vi "Get Device Name.vi"(8 "Error In":errorcluster, 11 "LINX Device Config":T1) -> (0 "Error Out":errorcluster, 2 "Device Name":string, 3 "LINX Device Config":T1)   [LabVIEW 2014, in "LMH-LINX.lvlib" / "Device.lvlib"]
uses:
  Device.lvlib
  Type Defs/LINX Device Config.ctl
  Type Defs/Interface.ctl
  Type Defs/TCP Config.ctl
  Type Defs/Channels.ctl
  Type Defs/Error Type.ctl
  LMH-LINX.lvlib
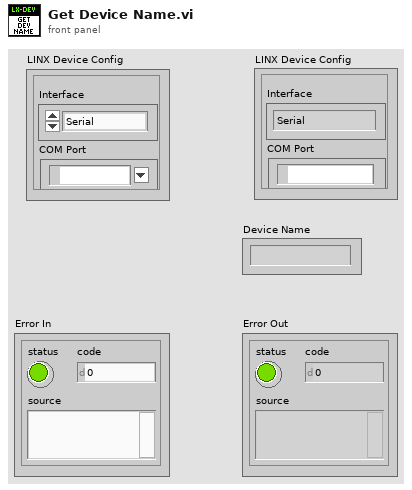
[diagram p1: front panel]
types:
  T1 = typedef "LMH-LINX.lvlib/Device.lvlib/LINX Device Config.ctl" = cluster{"Interface":T2, "COM Port":refnum<visa-resource-name>, "TCP Configuration":T3, "Device Family":u8, "Device ID":u8, "Device Name":string, "TCP Ref":refnum<k5>, "Channels":T4}
  T2 = typedef "LMH-LINX.lvlib/Interface.ctl" = enum16{"Serial", "TCP"}
  T3 = typedef "LMH-LINX.lvlib/Device.lvlib/TCP Config.ctl" = cluster{"IP Address":string, "Port":u16}
  T4 = typedef "LMH-LINX.lvlib/Channels.ctl" = cluster{"DI":u8[], "DO":u8[], "AI":u8[], "AO":u8[], "PWM":u8[], "QE":u8[], "UART":u8[], "I2C 2":u8[], "SPI":u8[], "CAN":u8[], "Servo":u8[], "AI Ref (V)":dbl, "AO Ref (V)":dbl, "AO Resolution (Bits)":u8}
  T5 = typedef "LMH-LINX.lvlib/Error Type.ctl" = enum16{"Unknown", "Timeout", "Corrupt Return Packet", "Unable To Connect", "Command Not Supported", "Channel DNE", "Invalid COM Config", "Firmware Version Mismatch", "myRIO Support", "CMD Specific Error"}
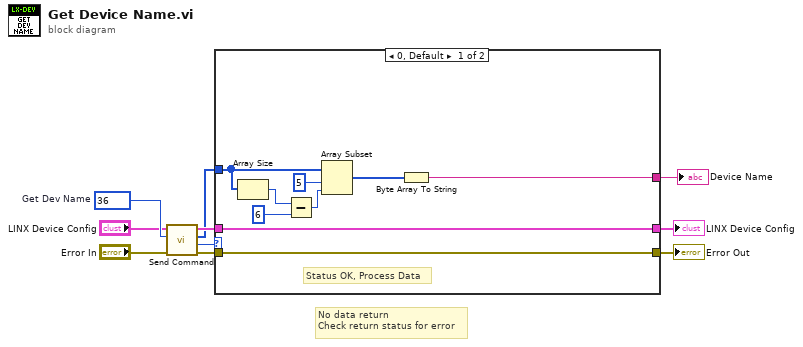
[diagram p0: block diagram]
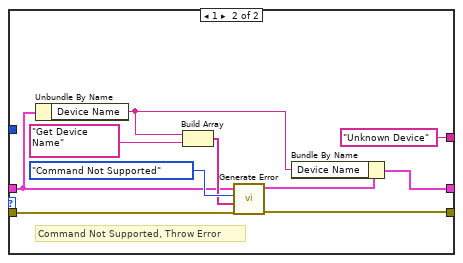
[diagram p2: hidden frame]
diagram:
  w9 = u16 36  # Get Dev Name
  # "No data return\nCheck return status for error"
  n1 = call "Send Command.vi"("Error In"="Error In", "CMD"=w9, "LINX Device Config"="LINX Device Config") -> ("Error Out"=w4:errorcluster, "Status"=w2:u8, "Response"=w3:u8[], "LINX Device Config"=w6:T1)  [unwired: 5 in]
  n2 = case shown="0, Default" w2 {
    tunnel: [w12 w23] -> w7
    tunnel: w6 -> [w12 w22]
    tunnel: [w11 w28] -> w5
    tunnel: w4 -> [w11 w29]
    tunnel: w3 -> [w19 _]
    tunnel: [w13 "Unknown Device" ("string")] -> w1
    frame 0, Default {
      # "Status OK, Process Data"
      n3 = Array Size(array=w19) -> (size(s)=w18:i32)
      n4 = Subtract(x=w18, y=6 ("index")) -> (x-y=w15:i32)
      n5 = Array Subset(array=w19, index=5, length=w15) -> (w14:u8[])
      n6 = Byte Array To String(unsigned byte array=w14) -> (string=w13:string)
    }
    frame 1 {
      # "Command Not Supported, Throw Error"
      n7 = Unbundle By Name(w22) -> ("Device Name"=w21:string)
      n8 = Build Array(w21, "Get Device Name") -> (w25:string[])
      n9 = call "Generate Error.vi"("Error In"=w29, "Arguments"=w25, "Error Type"=Error_Type."Command Not Supported", "LINX Device Config"=w22) -> ("Error Out"=w28:errorcluster, "Dup LINX Device Config"=w24:T1)  [unwired: 6 in]
      n10 = Bundle By Name(cluster=w24, "Device Name"=w21) -> (w23:T1)
    }
  }
  "Error Out" <- w5
  "LINX Device Config" <- w7
  "Device Name" <- w1
